vi "Write Com_Set.vi"(8 "error in (no error)":errorcluster, 10 "Com_Set":T1, 11 "TCP In":refnum<class "TCP.lvclass">) -> (0 "error out":errorcluster, 3 "TCP Out":refnum<class "TCP.lvclass">)   [LabVIEW 2019, in "TCP.lvclass"]
uses:
  TCP.lvclass
  SettingCtrl.ctl
  TCP.lvclass/TCP.ctl
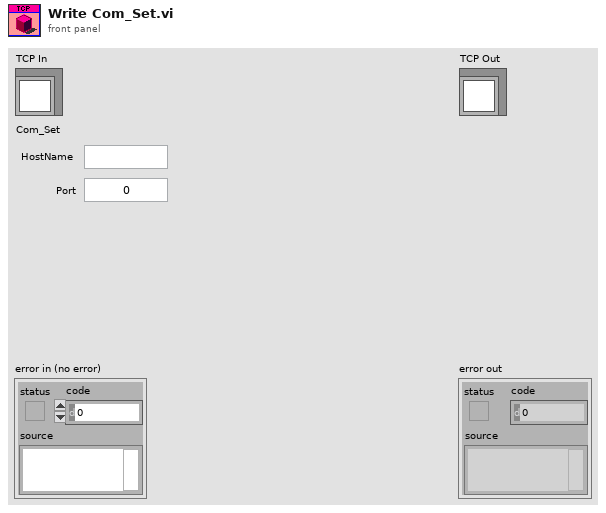
[diagram p1: front panel]
types:
  T1 = typedef "TCP.lvclass/SettingCtrl.ctl" = cluster{"HostName":string, "Port":u16}
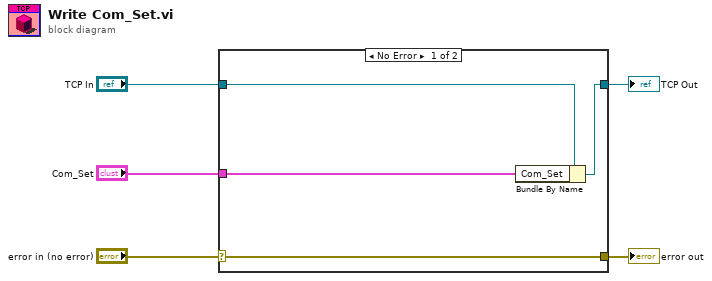
[diagram p0: block diagram]
diagram:
  n1 = case shown="No Error" "error in (no error)" {
    selector: "error in (no error)" -> [w9 w10]
    tunnel: [w9 w10] -> w4
    tunnel: [w7 w11] -> w2
    tunnel: "TCP In" -> [w8 w11]
    tunnel: "Com_Set" -> [w6 _]
    frame No Error {
      n2 = Bundle By Name(cluster=w8, "Com_Set"=w6) -> (w7:refnum<class "TCP.lvclass">)
    }
    frame Error {
    }
  }
  "error out" <- w4
  "TCP Out" <- w2
